vi "查看测试时间.vi"(11 "文件名":string) -> (0 "错误输出":errorcluster, 2 "最小值":timestamp, 3 "最大值":timestamp)   [LabVIEW 2014]
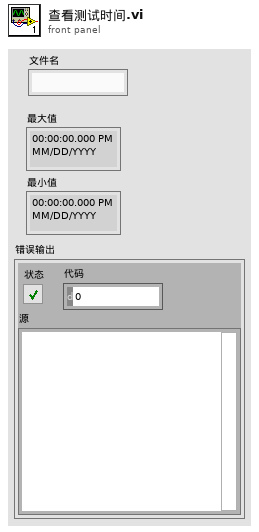
[diagram p1: front panel]
types:
  T1 = enum16{"open", "open or create", "create or replace", "create", "open (read-only)"}
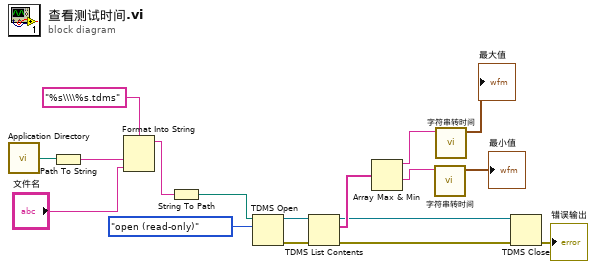
[diagram p0: block diagram]
diagram:
  n1 = call <vilib>:"Application Directory.vi"() -> ("Application Directory"=w17:path)
  n2 = Path To String(path=w17) -> (string=w15:string)
  n3 = Format Into String(format string="%s\\\\%s.tdms", w15, "文件名") -> (resulting string=w14:string)  [unwired: 2 in, 1 out]
  n4 = String To Path(string=w14) -> (path=w12:path)
  n5 = TDMS Open(10:T1."open (read-only)" ("操作(0:open)"), 11:w12) -> (0:w8:errorcluster, 3:w11:refnum<k34>)  [unwired: 5 in]
  n6 = TDMS List Contents(4:w8, 7:w11) -> (0:w5:errorcluster, 2:w9:string[], 3:w6:refnum<k34>)  [unwired: 1 in, 1 out]
  n7 = Array Max & Min(array=w9) -> (max value=w4:string, min value=w2:string)  [unwired: 2 out]
  n8 = call "字符串转时间.vi"("时间字符串"=w2) -> ("时间标识"=→"最小值":timestamp)  [unwired: 10 in]
  n9 = call "字符串转时间.vi"("时间字符串"=w4) -> ("时间标识"=→"最大值":timestamp)  [unwired: 10 in]
  n10 = TDMS Close(8:w5, 11:w6) -> (0:→"错误输出":errorcluster)  [unwired: 1 out]
